vi "Initialize.vi"(8 "error in":errorcluster, 11 "Plugin in":refnum<class "FFT.lvclass">) -> (0 "error out":errorcluster, 3 "Plugin out":refnum<class "FFT.lvclass">)   [LabVIEW 2024, in "FFT.lvlib" / "FFT.lvclass"]
uses:
  FFT.lvclass
  C:/Program Files/National Instruments/LabVIEW 2024/vi.lib/FlexLogger/SDK/PluginSDK.lvlibp/PEFClasses/SDK/Plugin/Plugin.lvclass
  <vilib>/FlexLogger/SDK/PluginSDK.lvlibp/PEFClasses/SDK/System Interface/Resampling Mode.ctl
  <vilib>/FlexLogger/SDK/PluginSDK.lvlibp/PEFClasses/SDK/Processing Element/Timing Parameters.ctl
  <vilib>/FlexLogger/SDK/PluginSDK.lvlibp/PEFClasses/SDK/Processing Element/Timing Method.ctl
  FFT.lvclass/FFT.ctl
  FFT Globals.vi
  <vilib>/FlexLogger/SDK/PluginSDK.lvlibp/PEFClasses/SDK/Plugin/ParameterAccess/Write N Channel.vi
  <vilib>/FlexLogger/SDK/PluginSDK.lvlibp/PEFClasses/SDK/Plugin/Plugin.lvclass
  <vilib>/FlexLogger/SDK/PluginSDK.lvlibp/PEFClasses/SDK/System Interface/System Interface.lvclass
  C:/Program Files/National Instruments/LabVIEW 2024/vi.lib/FlexLogger/SDK/PluginSDK.lvlibp/PEFClasses/SDK/Processing Element/Processing Element.lvclass
  C:/Users/Administrator/Documents/LabVIEW Projects/FlexLogger IO Plug-ins/FFT/FFT.lvclass
  <vilib>/FlexLogger/SDK/PluginSDK.lvlibp/PEFClasses/SDK/Processing Element/Processing Element.lvclass
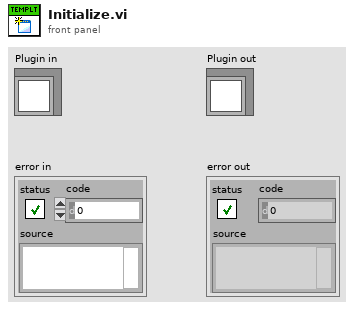
[diagram p1: front panel]
types:
  T1 = typedef "PluginSDK.lvlibp/Processing Element.lvclass/Timing Parameters.ctl" = cluster{"Timing Method":T2, "Timing Period (ms)":i32}
  T2 = typedef "PluginSDK.lvlibp/Processing Element.lvclass/Timing Method.ctl" = enum16{"Periodic", "Immediate", "On Data Ready", "Triggered"}
  T3 = typedef "PluginSDK.lvlibp/System Interface.lvclass/Resampling Mode.ctl" = enum16{"No Resampling", "Custom Rate", "Maximum Rate", "Minimum Rate"}
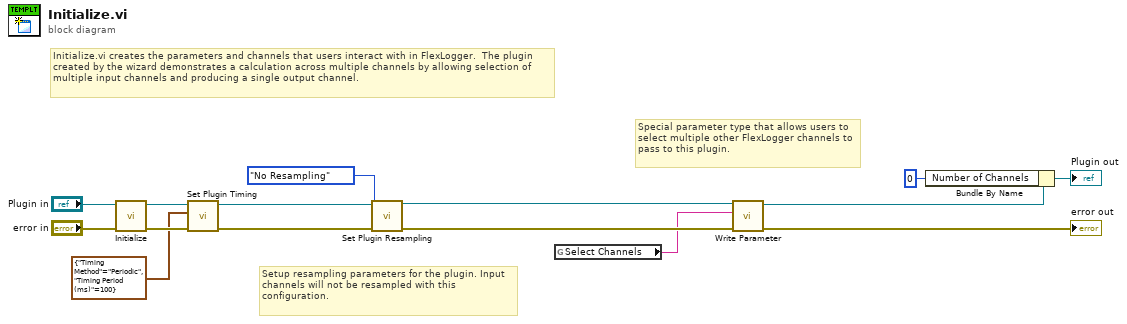
[diagram p0: block diagram]
diagram:
  # "Setup resampling parameters for the plugin. Input channels will not be resampled with this configuration."
  # "Special parameter type that allows users to select multiple other FlexLogger channels to pass to this plugin."
  # "Initialize.vi creates the parameters and channels that users interact with in FlexLogger.  The plugin created by the wizard demonstrates a calculation across multiple channels by allowing selection of multiple input channels and producing a single output channel."
  n1 = call-parent "Initialize.vi"("error in (no error)"="error in", "Plugin in"="Plugin in") -> ("error out"=w3:errorcluster, "Plugin out"=w5:refnum<class "FFT.lvclass">)  [unwired: 8 in]
  n2 = call <vilib>:"Set Plugin Timing.vi"("error in (no error)"=w3, "Timing Parameters"=T1 {"Timing Method"=enum."Periodic", "Timing Period (ms)"=100}, "Plugin in"=w5) -> ("error out"=w2:errorcluster, "Plugin out"=w4:refnum<class "FFT.lvclass">)  [unwired: 7 in]
  n3 = call <vilib>:"Set Plugin Resampling.vi"("Plugin in"=w4, "Resampling Mode"=Resampling_Mode."No Resampling", "error in (no error)"=w2) -> ("Plugin out"=w13:refnum<class "FFT.lvclass">, "error out"=w12:errorcluster)  [unwired: 11 in]
  n4 = global read "FFT Globals.vi" "Select Channels"() -> (w10:string)
  n5 = call-poly <vilib>:"Write Parameter.vi"("error in (no error)"=w12, "Name (Unique Channel Identifier)"=w10, "Plugin in"=w13) -> ("error out"=→"error out":errorcluster, "Plugin out"=w8:refnum<class "FFT.lvclass">)  [unwired: 7 in]
  n6 = Bundle By Name(cluster=w8, "Number of Channels"=0) -> (→"Plugin out":refnum<class "FFT.lvclass">)
